vi "Error Channels Write Array.vi"(8 "error in":errorcluster, 10 "Error Channels STS":i32[](array[numeric]), 11 "Cycler in":refnum<class "Cycler.lvclass">) -> (0 "error out":errorcluster, 3 "Cycler out":refnum<class "Cycler.lvclass">)   [LabVIEW 2023, in "Cycler.lvclass"]
uses:
  Cycler.lvclass
  Cycler.lvclass/Cycler.ctl
  Low Level Capabilities/Error Channels/Error Channels.lvclass
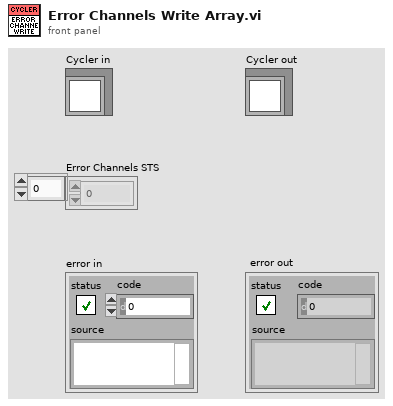
[diagram p1: front panel]
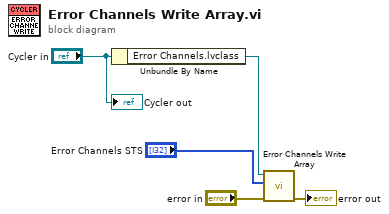
[diagram p0: block diagram]
diagram:
  n1 = Unbundle By Name("Cycler in") -> ("Error Channels.lvclass"=w5:refnum<class "Error Channels.lvclass">)
  n2 = call-dynamic "Error Channels Write Array.vi"("error in (no error)"="error in", "Error Channels STS"="Error Channels STS", "Error Channels in"=w5) -> ("error out"=→"error out":errorcluster)  [unwired: 7 in, 1 out]
  "Cycler out" <- "Cycler in"
